vi "FindUSB5DAQ.vi"(8 "错误输入（无错误）":errorcluster) -> (0 "error out":errorcluster caption="错误输出", 3 "DeviceCounts":i32)   [LabVIEW 2020]
uses:
  lib/x64/USB5000.dll
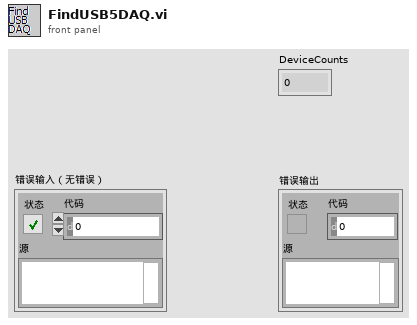
[diagram p1: front panel]
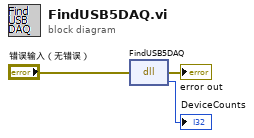
[diagram p0: block diagram]
diagram:
  n1 = dll-call lib="C:/Users/phosense/Downloads/USB-5000/usb5000_labview_cv/lib/x64/USB5000.dll" fn="FindUSB5DAQ"(error in="错误输入（无错误）") -> (error out=→"error out":errorcluster, "返回类型"=→"DeviceCounts":i32)  [unwired: 2 in, 1 out]
